vi "Traj.vi"(6 "error in":errorcluster, 7 "StartPos":dbl[](array[numeric]), 8 "Repeat number":i16, 9 "Acc":dbl, 10 "Vel":dbl, 11 "String":string) -> (2 "error out":errorcluster)   [LabVIEW 2022 SP3]
uses:
  Newport.XPS.CommandInterface
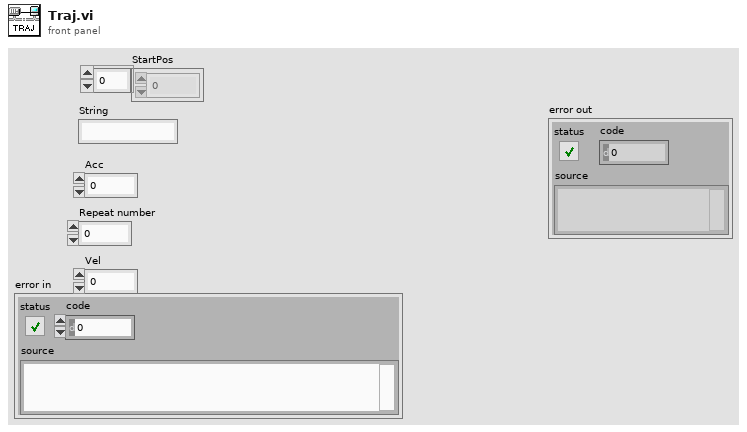
[diagram p1: front panel]
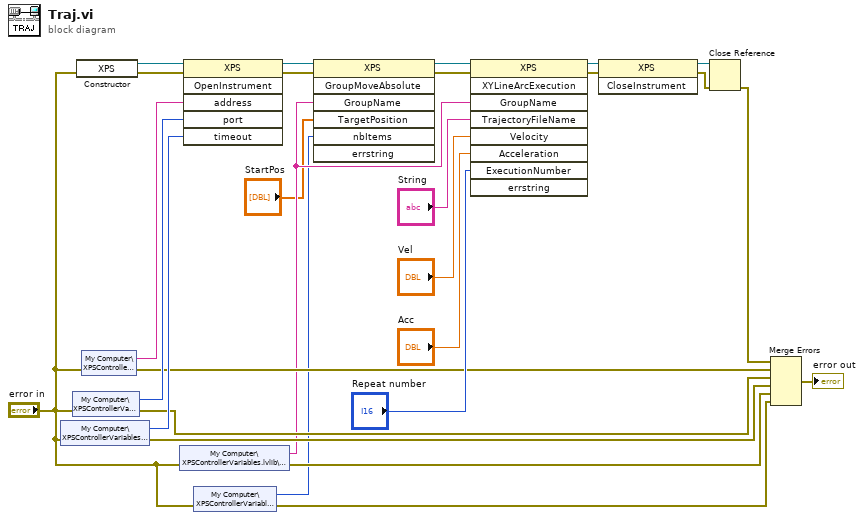
[diagram p0: block diagram]
diagram:
  n1 = shared-variable "My Computer\\XPSControllerVariables.lvlib\\Timeout"(error in="error in") -> (w24:i16, error out=w14:errorcluster)
  n2 = shared-variable "My Computer\\XPSControllerVariables.lvlib\\Port"(error in="error in") -> (w25:i16, error out=w15:errorcluster)
  n3 = constructor class="XPS"(error in="error in") -> (reference out=w28:refnum<k24>, error out=w27:errorcluster)  [unwired: 2 in, 1 out]
  n4 = shared-variable "My Computer\\XPSControllerVariables.lvlib\\IP"(error in="error in") -> (w26:string, error out=w16:errorcluster)
  n5 = shared-variable "My Computer\\XPSControllerVariables.lvlib\\GroupName"(error in="error in") -> (w5:string, error out=w13:errorcluster)
  n6 = invoke class="XPS" method="OpenInstrument"(reference=w28, error in=w27, "address"=w26, "port"=w25, "timeout"=w24) -> (reference out=w9:refnum<k24>, error out=w8:errorcluster)  [unwired: 1 in, 4 out]
  n7 = shared-variable "My Computer\\XPSControllerVariables.lvlib\\nbitem"(error in="error in") -> (w4:i16, error out=w2:errorcluster)
  n8 = invoke class="XPS" method="GroupMoveAbsolute"(reference=w9, error in=w8, "GroupName"=w5, "TargetPosition"="StartPos", "nbItems"=w4) -> (reference out=w7:refnum<k24>, error out=w6:errorcluster)  [unwired: 2 in, 5 out]
  n9 = invoke class="XPS" method="XYLineArcExecution"(reference=w7, error in=w6, "GroupName"=w5, "TrajectoryFileName"="String", "Velocity"="Vel", "Acceleration"="Acc", "ExecutionNumber"="Repeat number") -> (reference out=w20:refnum<k24>, error out=w19:errorcluster)  [unwired: 2 in, 7 out]
  n10 = invoke class="XPS" method="CloseInstrument"(reference=w20, error in=w19) -> (reference out=w18:refnum<k24>, error out=w17:errorcluster)  [unwired: 1 in, 1 out]
  n11 = Close Reference(reference=w18, error in (no error)=w17) -> (error out=w12:errorcluster)
  n12 = Merge Errors(w12, w16, w15, w14, w13, w2) -> (→"error out":errorcluster)
